vi "Receive.vi"(7 "Msg in":refnum<class "Msg.lvclass">, 11 "State in":refnum<class "State.lvclass">) -> (5 "Msg out":refnum<class "Msg.lvclass">)   [LabVIEW 2021, in "jettl.lvlib" / "State.lvclass"]
uses:
  State.lvclass
  Msg/Msg.lvclass
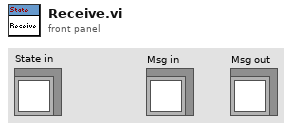
[diagram p1: front panel]
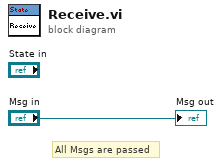
[diagram p0: block diagram]
diagram:
  # "All Msgs are passed"
  "Msg out" <- "Msg in"
